vi "Write DataSocket Configuration.vi"(8 "error in (no error)":errorcluster, 10 "Configuration":T1, 11 "DataSocket Client in":refnum<class "DataSocket Client.lvclass">) -> (0 "error out":errorcluster, 3 "DataSocket Client out":refnum<class "DataSocket Client.lvclass">)   [LabVIEW 2021, in "DataSocket Client.lvclass"]
uses:
  DataSocket Client.lvclass
  DataSocket Client.lvclass/DataSocket Client.ctl
  DataSocket Configuration.ctl
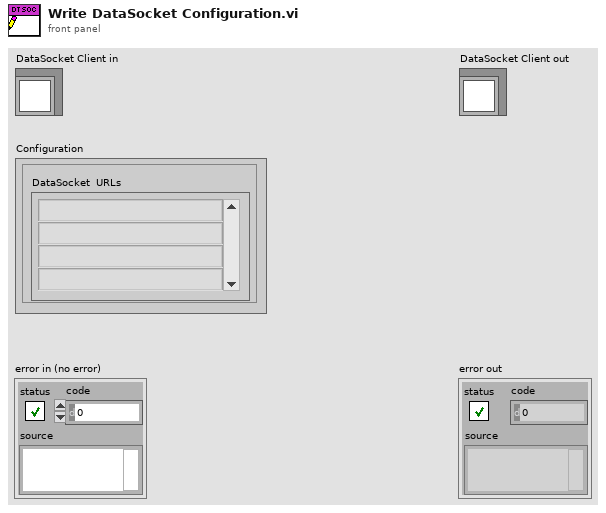
[diagram p1: front panel]
types:
  T1 = typedef "DataSocket Configuration.ctl" = cluster{"DataSocket  URLs":string[]}
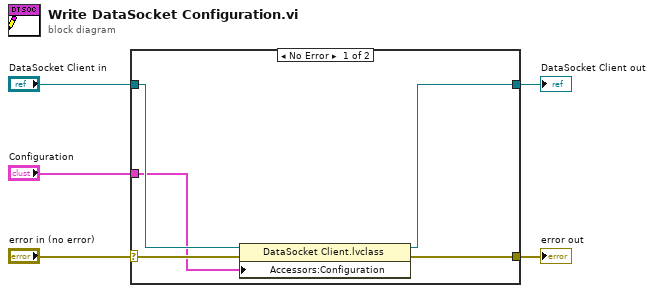
[diagram p0: block diagram]
diagram:
  n1 = case shown="No Error" "error in (no error)" {
    selector: "error in (no error)" -> [w10 w11]
    tunnel: [w9 w11] -> w4
    tunnel: [w7 w12] -> w2
    tunnel: "DataSocket Client in" -> [w8 w12]
    tunnel: "Configuration" -> [w6 _]
    frame No Error {
      n2 = property class="DataSocket Client.lvclass"(reference=w8, error in=w10, "Accessors:Configuration"=w6) -> (reference out=w7:refnum<class "DataSocket Client.lvclass">, error out=w9:errorcluster)
    }
    frame Error {
    }
  }
  "error out" <- w4
  "DataSocket Client out" <- w2
